vi "MessageName.vi"() -> (2 "MessageName":string)   [LabVIEW 2020, in "TcpAckNack.lvlib"]
uses:
  TcpAckNack.lvlib
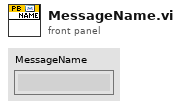
[diagram p1: front panel]
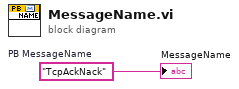
[diagram p0: block diagram]
diagram:
  w1 = "TcpAckNack"  # PB MessageName
  "MessageName" <- w1
